vi "Process TC Data.vi"(1 "TC Data Raw":dbl[](array[numeric])) -> (0 "TC Cluster":T1 {"TC 16" scale=0.0..100.0; "TC 15" scale=0.0..100.0; "TC 14" scale=0.0..100.0; "TC 13" scale=0.0..100.0; "TC 12" scale=0.0..100.0; "TC 11" scale=0.0..100.0; "TC 10" scale=0.0..100.0; "TC 9" scale=0.0..100.0; "TC 8" scale=0.0..100.0; "TC 7" scale=0.0..100.0; "TC 6" scale=0.0..100.0; "TC 5" scale=0.0..100.0; "TC 4" scale=0.0..100.0; "TC 3" scale=0.0..100.0; "TC 2" scale=0.0..100.0; "TC 1" scale=0.0..2.0})   [LabVIEW 2017]
uses:
  Controls/TC Indicator Cluster.ctl
  cRIO Convert Thermocouple Readings.llb/Thermocouple Type.ctl
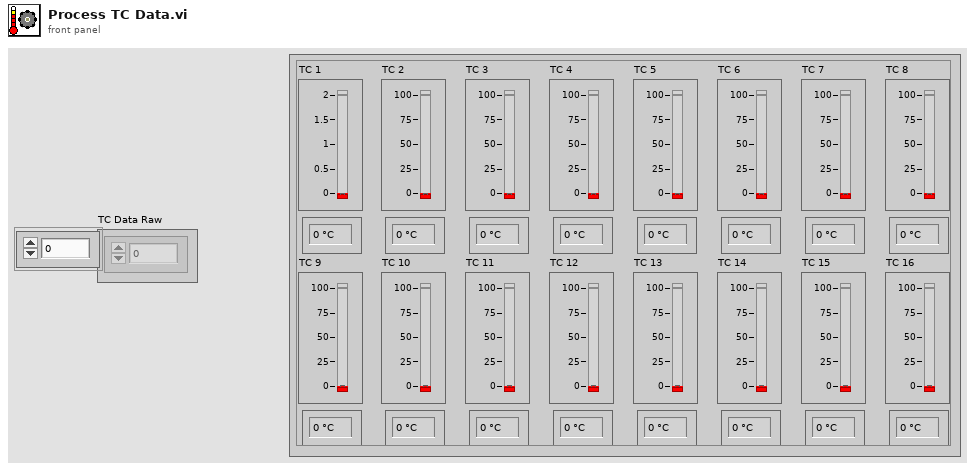
[diagram p1: front panel]
types:
  T1 = typedef "TC Indicator Cluster.ctl" = cluster{"TC 1":dbl, "TC 2":dbl, "TC 3":dbl, "TC 4":dbl, "TC 5":dbl, "TC 6":dbl, "TC 7":dbl, "TC 8":dbl, "TC 9":dbl, "TC 10":dbl, "TC 11":dbl, "TC 12":dbl, "TC 13":dbl, "TC 14":dbl, "TC 15":dbl, "TC 16":dbl}
  T2 = typedef "Thermocouple Type.ctl" = u16
  T3 = cluster{"[0]":dbl, "[1]":dbl, "[2]":dbl, "[3]":dbl, "[4]":dbl, "[5]":dbl, "[6]":dbl, "[7]":dbl, "[8]":dbl, "[9]":dbl, "[10]":dbl, "[11]":dbl, "[12]":dbl, "[13]":dbl, "[14]":dbl, "[15]":dbl}
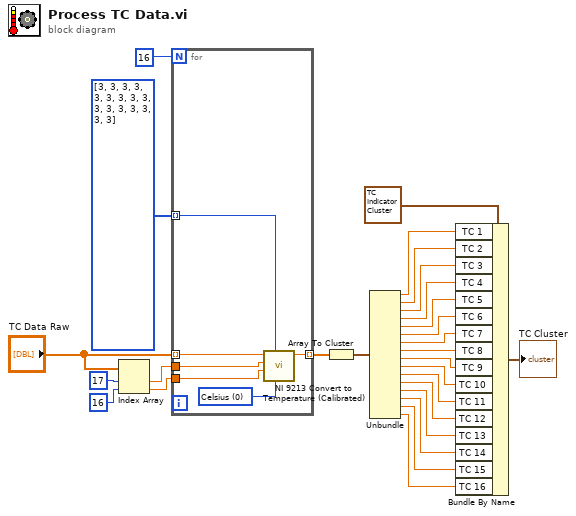
[diagram p0: block diagram]
diagram:
  w27 = T2[] [3, 3, 3, 3, 3, 3, 3, 3, 3, 3, 3, 3, 3, 3, 3, 3] items=["B", "E", "J", "K", "R", "S", "T", "N"] ("Array")
  n1 = Index Array(array="TC Data Raw", index #1=17 ("index"), index #2=16 ("index")) -> (element #1=w25:dbl, element #2=w24:dbl)
  n2 = for {
    N: 16 -> [_]
    tunnel: w27 -> [w33] mode=indexing
    tunnel: "TC Data Raw" -> [w29] mode=indexing
    tunnel: w25 -> [w30]
    tunnel: w24 -> [w31]
    tunnel: [w28] -> w18 mode=indexing
    w32 = u16 0 items=["Celsius", "Fahrenheit", "Kelvin", "Rankine"] ("Temperature Units (C)")
    n3 = call "NI 9213 Convert to Temperature (Calibrated).vi"("Temperature Units (C)"=w32, "ThermocoupleType"=w33, "AutoZero"=w31, "CJC"=w30, "TC Input"=w29) -> ("Thermocouple Temperature"=w28:dbl)  [unwired: 6 in]
  }
  n4 = Array To Cluster(array=w18) -> (cluster=w17:T3)
  n5 = Unbundle(w17) -> ("[0]"=w16:dbl, "[1]"=w15:dbl, "[2]"=w14:dbl, "[3]"=w13:dbl, "[4]"=w12:dbl, "[5]"=w11:dbl, "[6]"=w10:dbl, "[7]"=w9:dbl, "[8]"=w8:dbl, "[9]"=w7:dbl, "[10]"=w6:dbl, "[11]"=w5:dbl, "[12]"=w4:dbl, "[13]"=w3:dbl, "[14]"=w2:dbl, "[15]"=w1:dbl)
  n6 = Bundle By Name(cluster=T1 {"TC 1"=0.0, "TC 2"=0.0, "TC 3"=0.0, "TC 4"=0.0, "TC 5"=0.0, "TC 6"=0.0, "TC 7"=0.0, "TC 8"=0.0, "TC 9"=0.0, "TC 10"=0.0, "TC 11"=0.0, "TC 12"=0.0, "TC 13"=0.0, "TC 14"=0.0, "TC 15"=0.0, "TC 16"=0.0} ("TC Cluster 2"), "TC 1"=w16, "TC 2"=w15, "TC 3"=w14, "TC 4"=w13, "TC 5"=w12, "TC 6"=w11, "TC 7"=w10, "TC 8"=w9, "TC 9"=w8, "TC 10"=w7, "TC 11"=w6, "TC 12"=w5, "TC 13"=w4, "TC 14"=w3, "TC 15"=w2, "TC 16"=w1) -> (→"TC Cluster":T1)
